vi "Overwrite-all-hidden-params.vi"(8 "error in (no error)":errorcluster, 10 "Config params adv":T1={"Image border size"=1, "Framegrabber board"=0, "Framegrabber buffer"=1, "Camera config file"=path "Support files/camera-config.mcf", "Framegrabber DLL file"=path "C:/CameraVision/Configuration/camera-config.mcf"} {"Framegrabber buffer" min=1; "Framegrabber board" min=0; "Image border size" min=0}, 11 "Config. params. ref. in":refnum<data-value>) -> (0 "error out":errorcluster, 3 "Config. params. ref.":refnum<data-value>)   [LabVIEW 2013, in "CameraVision.lvlib" / "CV-Configuration.lvclass"]
uses:
  CV-Configuration.lvclass
  Configuration-parameters-advanced.ctl
  CV-Configuration.lvclass/CV-Configuration.ctl
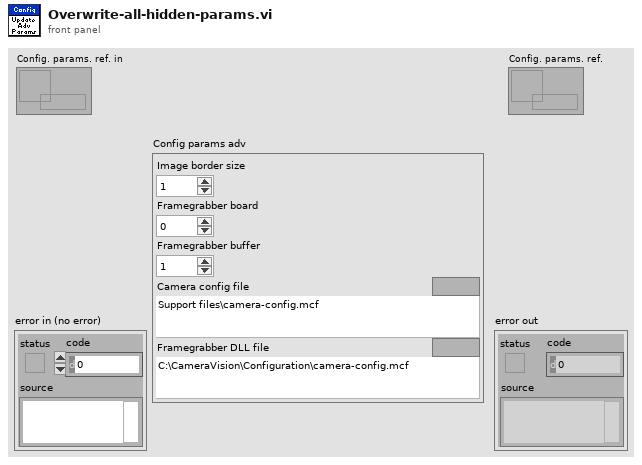
[diagram p1: front panel]
types:
  T1 = typedef "CameraVision.lvlib/CV-Configuration.lvclass/Configuration-parameters-advanced.ctl" = cluster{"Image border size":i32, "Framegrabber board":i32, "Framegrabber buffer":i32, "Camera config file":path, "Framegrabber DLL file":path}
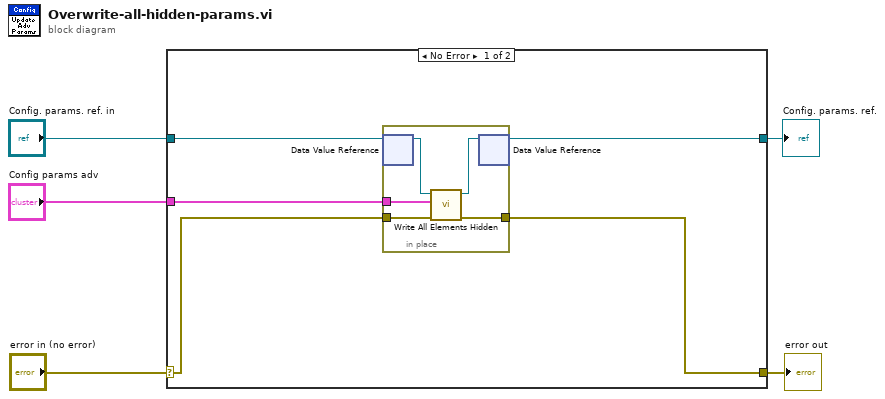
[diagram p0: block diagram]
diagram:
  n1 = case shown="No Error" "error in (no error)" {
    selector: "error in (no error)" -> [w8 w17]
    tunnel: [w9 w17] -> w4
    tunnel: "Config. params. ref. in" -> [w7 w16]
    tunnel: "Config params adv" -> [w10 _]
    tunnel: [w6 w16] -> w1
    frame No Error {
      n2 = in-place {
        in-place-border: w10 -> [w15]
        in-place-border: [w14] -> w9
        in-place-border: w8 -> [w13]
        n3 = in-place-dvr #1(w7) -> (w12:refnum<class "CV-Configuration.lvclass">)  [unwired: 1 out]
        n4 = call "Write All Elements Hidden.vi"("error in (no error)"=w13, "Config. params. hidden"=w15, "Config params in"=w12) -> ("error out"=w14:errorcluster, "Config params out"=w11:refnum<class "CV-Configuration.lvclass">)  [unwired: 7 in]
        n5 = in-place-dvr #1(w11) -> (w6:refnum<data-value>)  [unwired: 1 out]
      }
    }
    frame Error {
    }
  }
  "error out" <- w4
  "Config. params. ref." <- w1
